vi "MainV1.vi"() -> ()   [LabVIEW 2010]
uses:
  <vilib>/Instr/_visa.llb/VISA Set IO Buffer Mask.ctl
  <vilib>/Instr/_visa.llb/VISA Flush IO Buffer Mask.ctl
  GlobalVar.vi
  <vilib>/Instr/_visa.llb/VISA Configure Serial Port (Instr).vi
panel:
  out "LongToSend":u8
  out "TypeToSend":u8
  out "DataToSend":u8[](array[numeric])
  out "Frequency":dbl
  out "Enum":T1(ring)
  out "error":errorcluster
  out "error Connexion":errorcluster
  out "Stop main loop":bool
  in  "stop":bool
  in  "Tab Control":T2(tab)
  out "Comm_LEDTest":bool
  in  "Comm_TestConnection":bool
  in  "Comm_BaudRate":u32=9600 caption="Baud rate"
  in  "Comm_PortComm":refnum<visa-resource-name>="COM7" caption="Communication Port"
  in  "timeout (10sec)":u32=10000
  in  "Con_RefreshIntensity":bool caption="Bouton OK 12"
  in  "Con_RefreshRightTorque":bool caption="Bouton OK 12"
  out "Con_XYIntensity":cluster{"Y":dbl[], "Y":dbl[]}[](graph) caption="Intensity"
  out "Con_XYRightTorque":cluster{"Y":dbl[], "Y":dbl[]}[](graph) caption="Motor right Torque"
  in  "Con_RefreshLeftTorque":bool caption="Bouton OK 12"
  out "Con_XYLeftTorque":cluster{"Y":dbl[], "Y":dbl[]}[](graph) caption="Motor left Torque"
  out "Con_IntensityMax":bool caption="Max Intensity"
  out "Con_Intensity":string[][](array[string]) caption="Intensity (A)"
  out "Con_MotorRightTorque":string[][](array[string]) caption="Motor right Torque (N.m)"
  out "Con_MotorLeftTorque":string[][](array[string]) caption="Motor left Torque (N.m)"
  in  "Ana_RefreshBattery":bool caption="Bouton OK 12"
  out "Ana_XYBattery":cluster{"Y":dbl[], "Y":dbl[]}[](graph) caption="Motor left Torque"
  in  "Ana_RefreshHandlebar":bool caption="Bouton OK 12"
  out "Ana_XYHandlebar":cluster{"Y":dbl[], "Y":dbl[]}[](graph) caption="Motor left Torque"
  out "Ana_Battery":string[][](array[string]) caption="Battery"
  out "Ana_Handlebar":string[][](array[string]) caption="Handlebar"
  in  "Inc_RefreshAcceleration":bool caption="Bouton OK 12"
  out "Inc_XYAcceleration":cluster{"Y":dbl[], "Y":dbl[]}[](graph) caption="Motor left Torque"
  in  "Inc_RefreshVelocityRightMotor":bool caption="Bouton OK 12"
  out "Inc_XYVelocityRightMotor":cluster{"Y":dbl[], "Y":dbl[]}[](graph) caption="Motor left Torque"
  in  "Inc_RefreshVelocityLeftMotor":bool caption="Bouton OK 12"
  out "Inc_XYVelocityLeftMotor":cluster{"Y":dbl[], "Y":dbl[]}[](graph) caption="Motor left Torque"
  out "Inc_Acceleration":string[][](array[string]) caption="Acceleration"
  out "Inc_VelocityRightMotor":string[][](array[string]) caption="Velocity Right motor"
  out "Inc_VelocityLeftMotor":string[][](array[string]) caption="Velocity left motor"
  out "Other_AngularVelocity":string[][](array[string]) caption="Angular velocity"
  out "Other_AngleOUT":string[][](array[string]) caption="Angle Out of range"
  out "Other_SpeedSaturation":string[][](array[string]) caption="Speed saturation"
  out "Other_Distance":string[][](array[string]) caption="Distance"
  out "Other_Angle":string[][](array[string]) caption="Angle"
  out "Spe_XY":cluster{"Y":dbl[], "Y":dbl[]}[](graph) caption="Motor left Torque"
  in  "Spe_Time":dbl caption="Time"
  in  "Spe_SendAnalysis":bool caption="Send Analysis"
  in  "Spe_Frequency":dbl caption="Frequency"
  out "Spe_Liste":string(combo) caption="Type"
  in  "Config_VelocitySaturation":dbl caption="VelocitySaturation"
  in  "Config_Sendvelocitysaturation":bool caption="Set velocity saturation"
  out "Config_Ready":string caption="Ready"
  out "Config_CurrentState":string caption="Current state"
  in  "Config_SendReady":bool caption="Ready ?"
  in  "Config_SendCurrentState":bool caption="Current state ?"
  in  "Config_SendRestart":bool caption="Re Start system"
  in  "Config_SendSTOP":bool caption="STOP system"
  out "Config_tCoefKalman":dbl caption="tCoef Kalman"
  in  "Config_ReceiveKalman":bool
  in  "Config_SendCoefKalman":bool
  in  "Config_CoefKalman":dbl caption="Coef Kalman"
  in  "Config_SendCoefAcc":bool
  in  "Config_CoefAcc":dbl caption="Coef System Acc"
  out "Config_tCoefdir":dbl caption="tCoef direction"
  in  "Config_SendCoefDir":bool
  in  "Config_CoeffDir":dbl caption="Coeff dir"
  in  "Config_ReceiveCoefDir":bool
  out "Config_tD":dbl caption="tD"
  out "Config_tI":dbl caption="tI"
  out "Config_tK":dbl caption="tK"
  in  "Config_ReceiveD":bool caption="Bouton OK 6"
  in  "Config_ReceiveI":bool
  in  "Config_ReceiveK":bool
  in  "Config_SendD":bool
  in  "Config_SendI":bool
  in  "Config_SendK":bool
  in  "Config_D":dbl caption="D"
  in  "Config_I":dbl caption="I"
  in  "Config_K":dbl caption="K"
  in  "Config_SendPID":bool
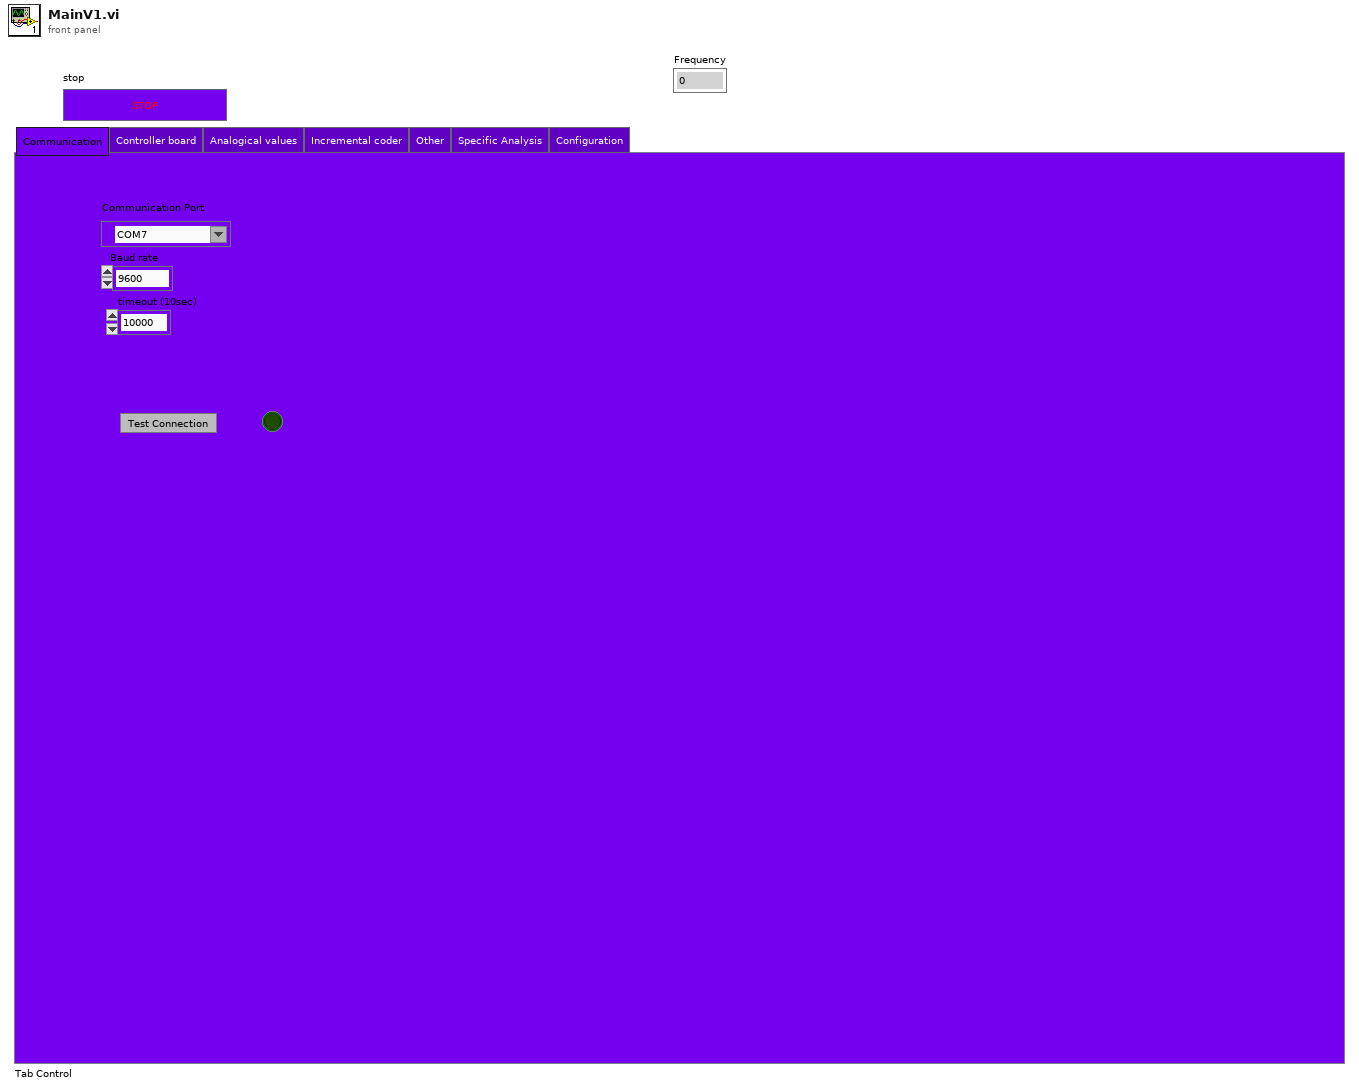
[diagram p1: front panel]
types:
  T1 = enum16{"Comm_TestConnection", "Con_RefreshLeftTorque", "Con_RefreshRightTorque", "Con_RefreshIntensity", "Ana_RefreshBattery", "Ana_RefreshHandlebar", "Inc_RefreshVelocityLeftMotor", "Inc_RefreshVelocityRightMotor", "Inc-RefreshAcceleration", "Spe_SendAnalysis", "Config_SendK", "Config_ReceiveK", "Config_SendD", "Config_ReceiveD", "Config_SendI", "Config_ReceiveI", "Config_SendCoefDir", "Config_ReceiveCoefDir", "Config_SendPID", "Config_SendCoefAcc", "Config_SendCoefKalman", "Config_ReceiveKalman", "Config_SendSTOP", "Config_SendRestart", "Config_SendCurrentState", "Config_SendReady", "Config_Sendvelocitysaturation", "Waiting"}
  T2 = enum32{"Communication", "Controller board", "Analogical values", "Incremental coder", "Other", "Specific Analysis", "Configuration"}
  T3 = typedef "VISA Set IO Buffer Mask.ctl" = u16
  T4 = typedef "VISA Flush IO Buffer Mask.ctl" = u16
  T5 = enum8{"Enabled", "Disabled", "Disabled and Grayed Out"}
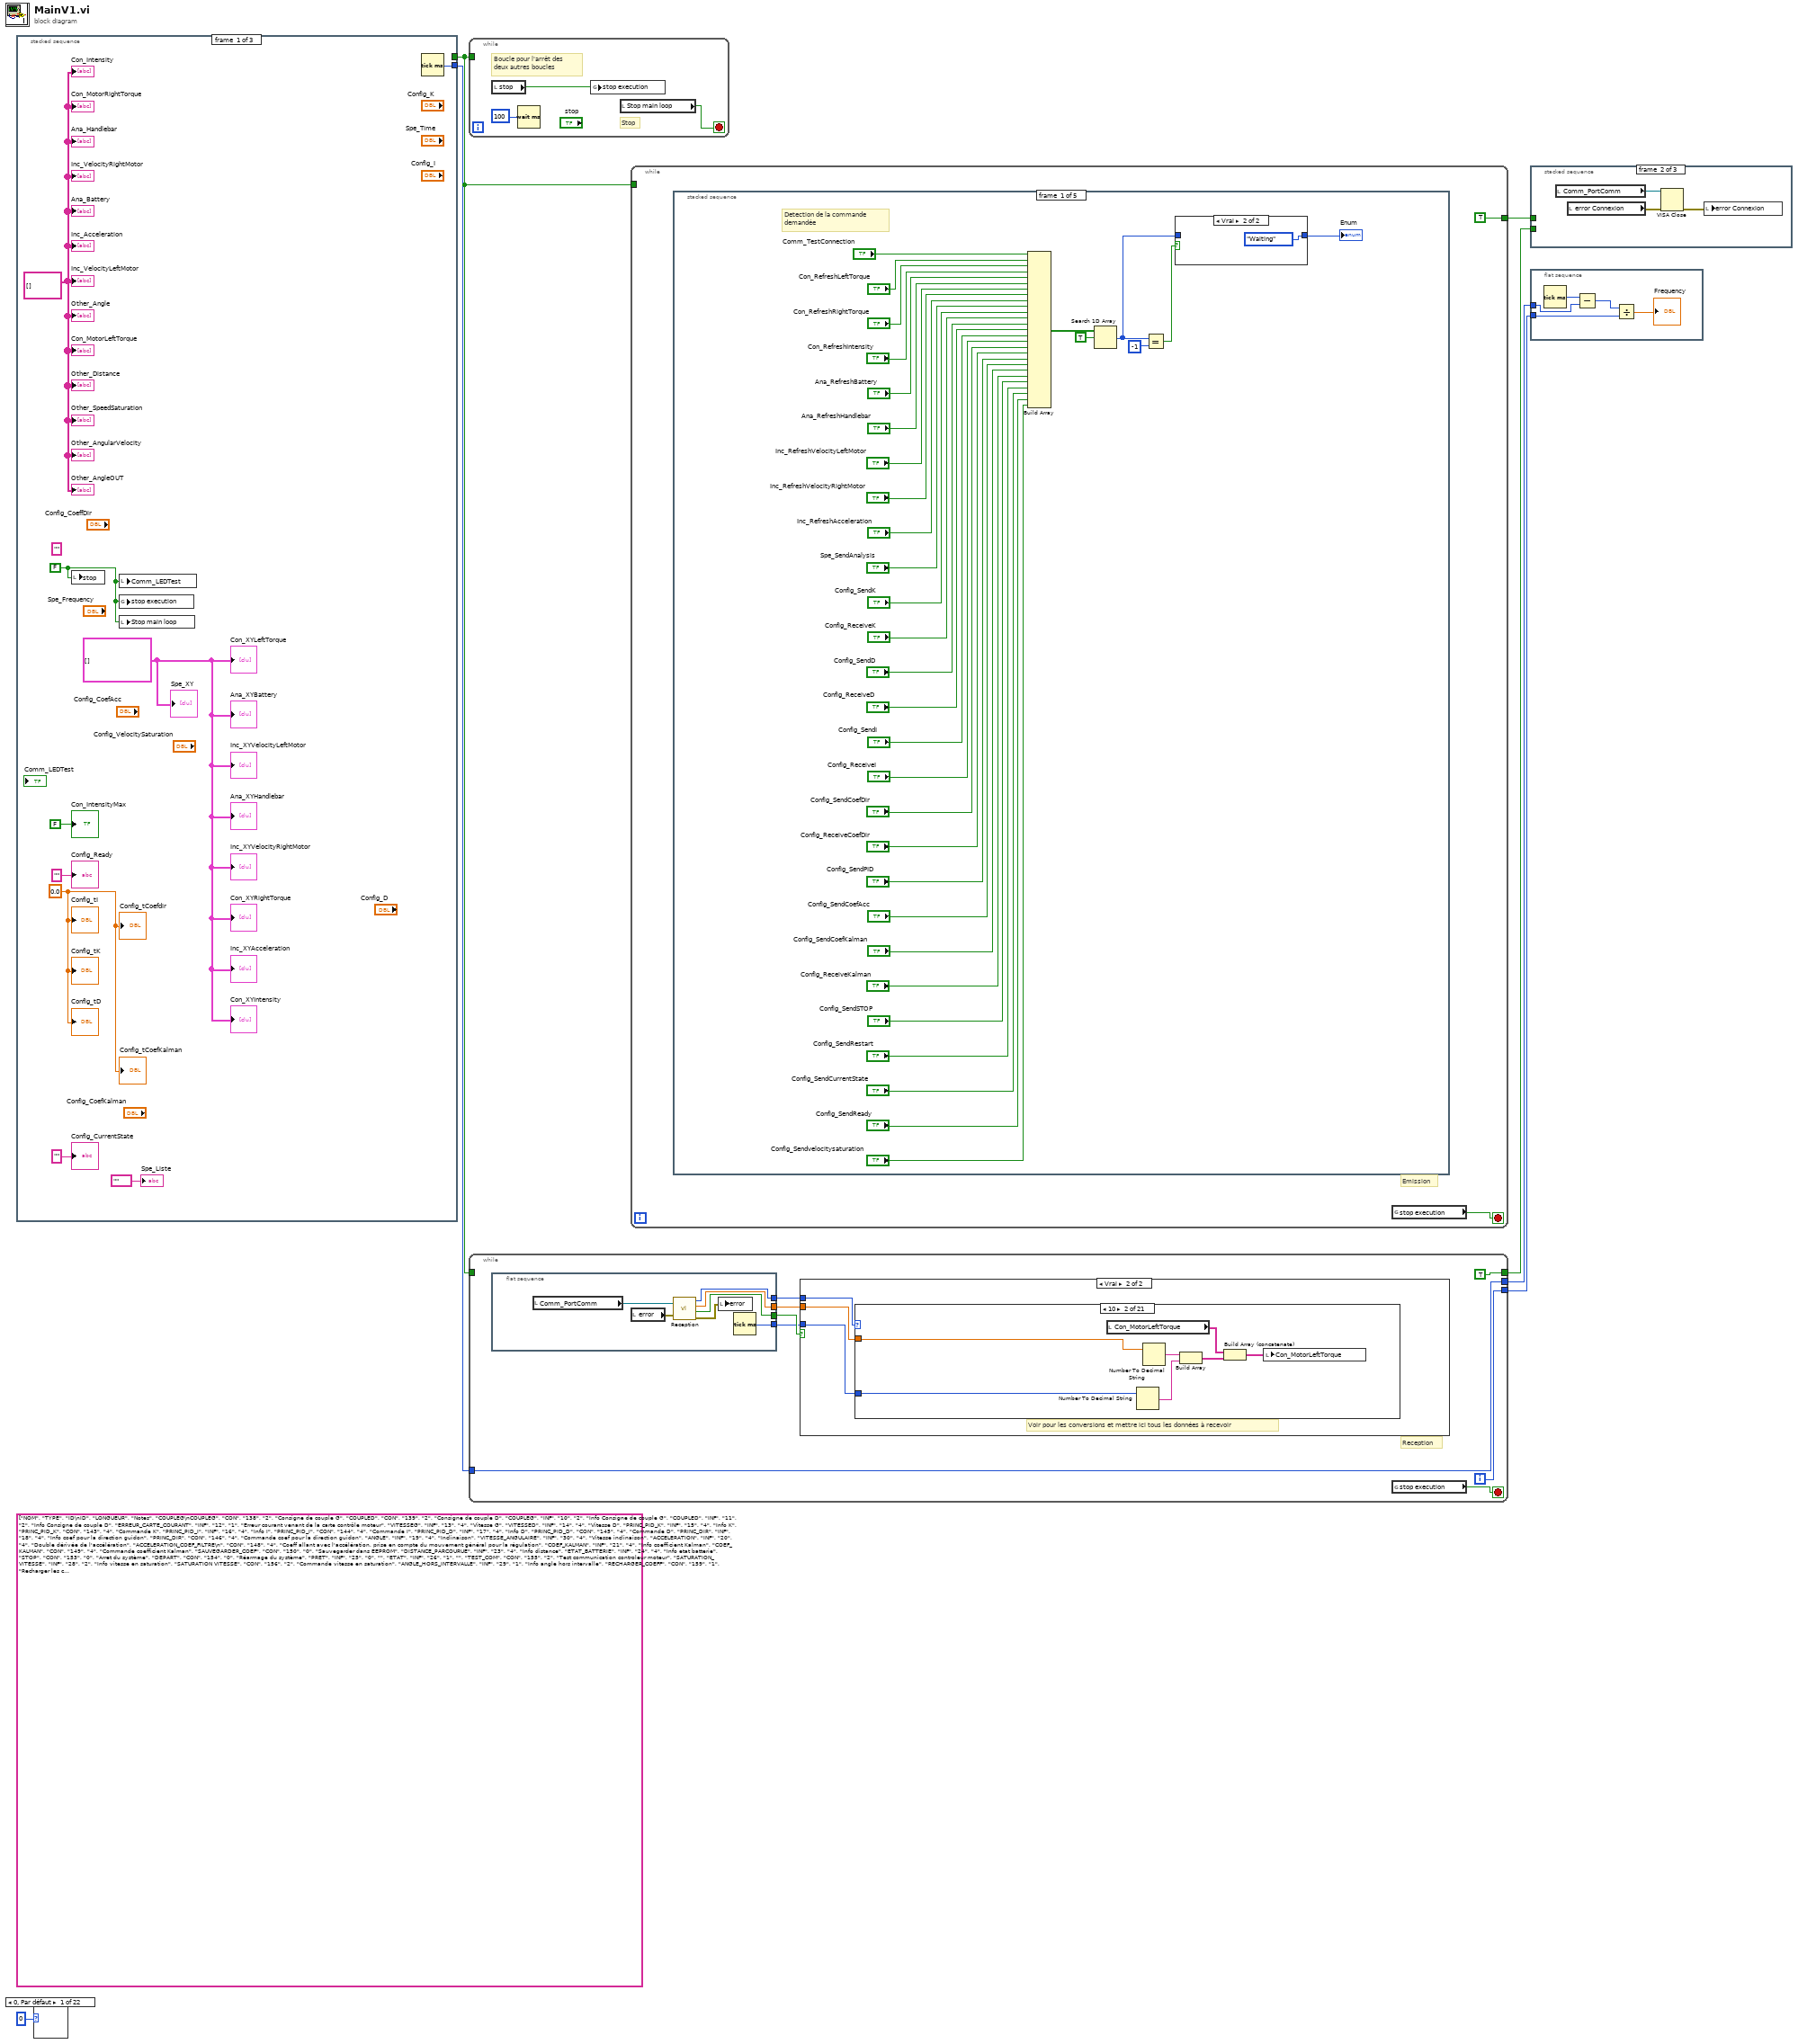
[diagram p0: block diagram]
diagram:
  (unwired) string[][] [["NOM", "TYPE", "ID\nID", "LONGUEUR", "Notes"], ["COUPLEG\nCOUPLEG", "CON", "138", "2", "Consigne de couple G"], ["COUPLED", "CON", "139", "2", "Consigne de couple D"], ["COUPLEG", "INF", "10", "2", "Info Consigne de couple G"], ["COUPLED", "INF", "11", "2", "Info Consigne de couple D"], ["ERREUR_CARTE_COURANT", "INF", "12", "1", "Erreur courant venant de la carte contrôle moteur"], ["VITESSEG", "INF", "13", "4", "Vitesse G"], ["VITESSED", "INF", "14", "4", "Vitesse D"], ["PRINC_PID_K", "INF", "15", "4", "Info K"], ["PRINC_PID_K", "CON", "143", "4", "Commande K"], ["PRINC_PID_I", "INF", "16", "4", "Info I"], ["PRINC_PID_I", "CON", "144", "4", "Commande I"], ["PRINC_PID_D", "INF", "17", "4", "Info D"], ["PRINC_PID_D", "CON", "145", "4", "Commande D"], ["PRINC_DIR", "INF", "18", "4", "Info coef pour la direction guidon"], ["PRINC_DIR", "CON", "146", "4", "Commande coef pour la direction guidon"], ["ANGLE", "INF", "19", "4", "Inclinaison"], ["VITESSE_ANGULAIRE", "INF", "30", "4", "Vitesse inclinaison"], ["ACCELERATION", "INF", "20", "4", "Double dérivée de l'accélération"], ["ACCELERATION_COEF_FILTRE\n", "CON", "148", "4", "Coeff allant avec l'accélération, prise en compte du mouvement général pour la régulation"], ["COEF_KALMAN", "INF", "21", "4", "Info coefficient Kalman"], ["COEF_KALMAN", "CON", "149", "4", "Commande coefficient Kalman"], ["SAUVEGARDER_COEF", "CON", "150", "0", "Sauvegarder dans EEPROM"], ["DISTANCE_PARCOURUE", "INF", "23", "4", "Info distance"], ["ETAT_BATTERIE", "INF", "24", "4", "Info etat batterie"], ["STOP", "CON", "153", "0", "Arret du système"], ["DEPART", "CON", "154", "0", "Réarmage du système"], ["PRET", "INF", "25", "0", ""], ["ETAT", "INF", "26", "1", ""], ["TEST_COM", "CON", "155", "2", "Test communication controleur moteur"], ["SATURATION_VITESSE", "INF", "28", "2", "Info vitesse en saturation"], ["SATURATION VITESSE", "CON", "156", "2", "Commande vitesse en saturation"], ["ANGLE_HORS_INTERVALLE", "INF", "29", "1", "Info angle hors intervalle"], ["RECHARGER_COEFF", "CON", "159", "1", "Recharger les coeff"]]
  n1 = stacked-sequence {
    tunnel: [_ _ TRUE] -> w7
    tunnel: [w15 _ _] -> w3
    frame #0 {
      w11 = 0.0 ("Config_tK")
      (unwired) "" ("Comm_Reception")
      w9 = cluster{"Y":dbl[], "Y":dbl[]}[] [] ("Ana_XYHandlebar 3")
      w8 = string[][] [] ("Velocity motor left")
      w16 = FALSE ("Comm_LEDTest")
      n2 = local write "stop"(w16) -> ()
      n3 = local write "Comm_LEDTest"(w16) -> ()
      n4 = global write "GlobalVar.vi" "stop execution"(w16) -> ()
      n5 = local write "Stop main loop"(w16) -> ()
      n6 = Tick Count (ms)() -> (millisecond timer value=w15:u32)
      "Con_IntensityMax" <- FALSE ("Con_IntensityMax")
      "Config_tK" <- w11
      "Config_tI" <- w11
      "Config_tD" <- w11
      "Config_tCoefdir" <- w11
      "Inc_Acceleration" <- w8
      "Config_tCoefKalman" <- w11
      "Other_Angle" <- w8
      "Config_CurrentState" <- "" ("Config_CurrentState")
      "Config_Ready" <- "" ("Config_Ready")
      "Other_SpeedSaturation" <- w8
      "Other_AngleOUT" <- w8
      "Other_Distance" <- w8
      "Ana_XYHandlebar" <- w9
      "Ana_XYBattery" <- w9
      "Inc_XYVelocityLeftMotor" <- w9
      "Inc_XYVelocityRightMotor" <- w9
      "Inc_XYAcceleration" <- w9
      "Spe_XY" <- w9
      "Con_MotorLeftTorque" <- w8
      "Con_MotorRightTorque" <- w8
      "Con_Intensity" <- w8
      "Inc_VelocityLeftMotor" <- w8
      "Inc_VelocityRightMotor" <- w8
      "Spe_Liste" <- "" ("Spe_Liste")
      "Ana_Handlebar" <- w8
      "Ana_Battery" <- w8
      "Con_XYRightTorque" <- w9
      "Con_XYIntensity" <- w9
      "Con_XYLeftTorque" <- w9
      "Other_AngularVelocity" <- w8
    }
    frame #1 {
      w18 = T3 48 items=["Buffer d'entrées (E/S)"=16, "Buffer de sorties (E/S)"=32, "Buffer d'entrées et de sorties (E/S)"=48] ("Mask")
      w22 = T4 16 items=["Vider le buffer d'entrées"=16, "Écrire le buffer de sorties sur le périphérique"=32, "Vider le buffer d'entrées (Pas d'E/S)"=64, "Vider le buffer de sorties"=128] ("Mask")
      w26 = u16 0 items=["None"=0, "XON/XOFF"=1, "RTS/CTS"=2, "DTR/DSR"=4] ("flow control")
      w27 = u16 10 items=["1.0"=10, "1.5"=15, "2.0"=20] ("stop bits")
      w29 = u16 0 items=["None", "Odd", "Even", "Mark", "Space"] ("parity")
      # "Initial"
      n7 = local write "Tab Control"(T2."Communication" ("Tab Control")) -> ()
      n8 = call-poly "VISA Configure Serial Port"("VISA resource name"="Comm_PortComm", "timeout (10sec)"="timeout (10sec)", "baud rate (9600)"="Comm_BaudRate", "data bits (8)"=u16 8 ("data bits"), "parity (0:none)"=w29, "stop bits (10: 1 bit)"=w27, "flow control (0:none)"=w26) -> ("VISA resource name out"=w23:refnum<visa-resource-name>, "error out"=w20:errorcluster)  [unwired: 2 in, 5 out]
      "error Connexion" <- w20
      "error" <- w20
      n9 = VISA Set I/O Buffer Size(VISA resource name=w23, mask (16)=w18, size (4096)=u32 524288 ("taille (4096)"), error in (no error)=w20) -> (VISA resource name out=w21:refnum<visa-resource-name>, error out=w19:errorcluster)
      n10 = VISA Flush I/O Buffer(VISA resource name=w21, mask (16)=w22, error in (no error)=w19) -> ()  [unwired: 2 out]
    }
    frame #2 {
      # "OK Initialisation"
    }
  }
  n11 = case shown="0, Par défaut" 0 {
    frame 0, Default {
    }
    frame 10 {
    }
    frame 11 {
    }
    frame 12 {
    }
    frame 13 {
    }
    frame 14 {
    }
    frame 15 {
    }
    frame 16 {
    }
    frame 17 {
    }
    frame 18 {
    }
    frame 19 {
    }
    frame 20 {
    }
    frame 21 {
    }
    frame 22 {
    }
    frame 23 {
    }
    frame 24 {
    }
    frame 25 {
    }
    frame 26 {
    }
    frame 27 {
    }
    frame 28 {
    }
    frame 29 {
    }
    frame 30 {
    }
  }
  n12 = while {
    tunnel: w7 -> [_]
    stop <- w34 stop-if-true
    # "Boucle pour l'arrêt des \ndeux autres boucles"
    # "Stop"
    n13 = local read "stop"() -> (w35:bool)
    n14 = Wait (ms)(milliseconds to wait=u32 100) -> ()  [unwired: 1 out]
    n15 = global write "GlobalVar.vi" "stop execution"(w35) -> ()
    n16 = local read "Stop main loop"() -> (w34:bool)
  }
  n17 = while {
    tunnel: w7 -> [_]
    tunnel: [TRUE] -> w6
    tunnel: w3 -> [w36]
    tunnel: [w37] -> w2
    tunnel: [w36] -> w1
    i -> [w37]
    stop <- w42 stop-if-true
    # "Reception"
    n18 = flat-sequence {
      tunnel: [w48] -> w41
      tunnel: [w47] -> w40
      tunnel: [w46] -> w39
      tunnel: [w45] -> w38
      frame #0 {
        n19 = local read "Comm_PortComm"() -> (w50:refnum<visa-resource-name>)
        n20 = local read "error"() -> (w49:errorcluster)
        n21 = call "Reception.vi"("entrée d'erreur (pas d'erreur)"=w49, "Nom de ressource VISA"=w50) -> ("Sortie d'erreur"=w44:errorcluster, "Checksum OK?"=w48:bool, "Data"=w46:dbl, "ID byte"=w47:i32)
        n22 = local write "error"(w44) -> ()
        n23 = Tick Count (ms)() -> (millisecond timer value=w45:u32)
      }
    }
    n24 = case shown="Vrai" w41 {
      tunnel: w40 -> [_ w53]
      tunnel: w39 -> [_ w52]
      tunnel: w38 -> [_ w51]
      frame False {
      }
      frame True {
        # "Voir pour les conversions et mettre ici tous les données à recevoir"
        n25 = case shown="10" w53 {
          tunnel: w52 -> [_ w59 w62 w69 w71 w79 w86 w87 w88 w89 w90 w99 w106 w108 w116 _ _ _ w124 _ w132]
          tunnel: w51 -> [_ w58 w61 _ w72 w80 _ _ _ _ w91 w98 _ w107 w115 _ _ _ w123 _ w131]
          frame 0, Default {
          }
          frame 10 {
            n26 = local read "Con_MotorLeftTorque"() -> (w60:string[][])
            n27 = Number To Decimal String(number=w58) -> (decimal integer string=w56:string)  [unwired: 1 in]
            n28 = Number To Decimal String(number=w59) -> (decimal integer string=w57:string)  [unwired: 1 in]
            n29 = Build Array(w57, w56) -> (w55:string[])
            n30 = Build Array (concatenate)(w60, w55) -> (w54:string[][])
            n31 = local write "Con_MotorLeftTorque"(w54) -> ()
          }
          frame 11 {
            n32 = local read "Con_MotorRightTorque"() -> (w67:string[][])
            n33 = Number To Decimal String(number=w61) -> (decimal integer string=w65:string)  [unwired: 1 in]
            n34 = Number To Decimal String(number=w62) -> (decimal integer string=w66:string)  [unwired: 1 in]
            n35 = Build Array(w66, w65) -> (w64:string[])
            n36 = Build Array (concatenate)(w67, w64) -> (w63:string[][])
            n37 = local write "Con_MotorRightTorque"(w63) -> ()
          }
          frame 12 {
            n38 = Not Equal To 0?(x=w69) -> (x != 0?=w68:bool)
            n39 = local write "Con_IntensityMax"(w68) -> ()
          }
          frame 13 {
            n40 = local read "Inc_VelocityLeftMotor"() -> (w77:string[][])
            n41 = Number To Decimal String(number=w72) -> (decimal integer string=w75:string)  [unwired: 1 in]
            n42 = Number To Exponential String(number=w71, precision (6)=i16 3 ("précision (6)")) -> (E-format string=w76:string)  [unwired: 2 in]
            n43 = Build Array(w76, w75) -> (w74:string[])
            n44 = Build Array (concatenate)(w77, w74) -> (w73:string[][])
            n45 = local write "Inc_VelocityLeftMotor"(w73) -> ()
          }
          frame 14 {
            n46 = local read "Inc_VelocityRightMotor"() -> (w85:string[][])
            n47 = Number To Decimal String(number=w80) -> (decimal integer string=w83:string)  [unwired: 1 in]
            n48 = Number To Exponential String(number=w79, precision (6)=i16 3 ("précision (6)")) -> (E-format string=w84:string)  [unwired: 2 in]
            n49 = Build Array(w84, w83) -> (w82:string[])
            n50 = Build Array (concatenate)(w85, w82) -> (w81:string[][])
            n51 = local write "Inc_VelocityRightMotor"(w81) -> ()
          }
          frame 15 {
            n52 = local write "Config_tK"(w86) -> ()
          }
          frame 16 {
            n53 = local write "Config_tI"(w87) -> ()
          }
          frame 17 {
            n54 = local write "Config_tD"(w88) -> ()
          }
          frame 18 {
            n55 = local write "Config_tCoefdir"(w89) -> ()
          }
          frame 19 {
            n56 = Number To Decimal String(number=w91) -> (decimal integer string=w95:string)  [unwired: 1 in]
            n57 = Number To Exponential String(number=w90, precision (6)=i16 3 ("précision (6)")) -> (E-format string=w96:string)  [unwired: 2 in]
            n58 = local read "Other_Angle"() -> (w97:string[][])
            n59 = Build Array(w96, w95) -> (w94:string[])
            n60 = Build Array (concatenate)(w97, w94) -> (w93:string[][])
            n61 = local write "Other_Angle"(w93) -> ()
          }
          frame 20 {
            n62 = local read "Inc_Acceleration"() -> (w105:string[][])
            n63 = Number To Decimal String(number=w98) -> (decimal integer string=w103:string)  [unwired: 1 in]
            n64 = Number To Exponential String(number=w99, precision (6)=i16 3 ("précision (6)")) -> (E-format string=w104:string)  [unwired: 2 in]
            n65 = Build Array(w104, w103) -> (w102:string[])
            n66 = Build Array (concatenate)(w105, w102) -> (w101:string[][])
            n67 = local write "Inc_Acceleration"(w101) -> ()
          }
          frame 21 {
            n68 = local write "Config_tCoefKalman"(w106) -> ()
          }
          frame 23 {
            n69 = Number To Decimal String(number=w107) -> (decimal integer string=w112:string)  [unwired: 1 in]
            n70 = local read "Other_Distance"() -> (w114:string[][])
            n71 = Number To Exponential String(number=w108, precision (6)=i16 3 ("précision (6)")) -> (E-format string=w113:string)  [unwired: 2 in]
            n72 = Build Array(w113, w112) -> (w111:string[])
            n73 = Build Array (concatenate)(w114, w111) -> (w110:string[][])
            n74 = local write "Other_Distance"(w110) -> ()
          }
          frame 24 {
            n75 = Number To Decimal String(number=w115) -> (decimal integer string=w120:string)  [unwired: 1 in]
            n76 = Number To Exponential String(number=w116, precision (6)=i16 3 ("précision (6)")) -> (E-format string=w121:string)  [unwired: 2 in]
            n77 = local read "Ana_Battery"() -> (w122:string[][])
            n78 = Build Array(w121, w120) -> (w119:string[])
            n79 = Build Array (concatenate)(w122, w119) -> (w118:string[][])
            n80 = local write "Ana_Battery"(w118) -> ()
          }
          frame 25 {
          }
          frame 26 {
          }
          frame 27 {
          }
          frame 28 {
            n81 = local read "Other_SpeedSaturation"() -> (w130:string[][])
            n82 = Number To Decimal String(number=w123) -> (decimal integer string=w128:string)  [unwired: 1 in]
            n83 = Number To Exponential String(number=w124, precision (6)=i16 3 ("précision (6)")) -> (E-format string=w129:string)  [unwired: 2 in]
            n84 = Build Array(w129, w128) -> (w127:string[])
            n85 = Build Array (concatenate)(w130, w127) -> (w126:string[][])
            n86 = local write "Other_SpeedSaturation"(w126) -> ()
          }
          frame 29 {
          }
          frame 30 {
            n87 = local read "Other_AngularVelocity"() -> (w138:string[][])
            n88 = Number To Decimal String(number=w131) -> (decimal integer string=w136:string)  [unwired: 1 in]
            n89 = Number To Exponential String(number=w132, precision (6)=i16 3 ("précision (6)")) -> (E-format string=w137:string)  [unwired: 2 in]
            n90 = Build Array(w137, w136) -> (w135:string[])
            n91 = Build Array (concatenate)(w138, w135) -> (w134:string[][])
            n92 = local write "Other_AngularVelocity"(w134) -> ()
          }
        }
      }
    }
    n93 = global read "GlobalVar.vi" "stop execution"() -> (w42:bool)
  }
  n94 = while {
    tunnel: w7 -> [_]
    tunnel: [TRUE] -> w5
    stop <- w139 stop-if-true
    # "Emission"
    n95 = stacked-sequence {
      frame #0 {
        # "Detection de la commande\ndemandée"
        n96 = Build Array("Comm_TestConnection", "Con_RefreshLeftTorque", "Con_RefreshRightTorque", "Con_RefreshIntensity", "Ana_RefreshBattery", "Ana_RefreshHandlebar", "Inc_RefreshVelocityLeftMotor", "Inc_RefreshVelocityRightMotor", "Inc_RefreshAcceleration", "Spe_SendAnalysis", "Config_SendK", "Config_ReceiveK", "Config_SendD", "Config_ReceiveD", "Config_SendI", "Config_ReceiveI", "Config_SendCoefDir", "Config_ReceiveCoefDir", "Config_SendPID", "Config_SendCoefAcc", "Config_SendCoefKalman", "Config_ReceiveKalman", "Config_SendSTOP", "Config_SendRestart", "Config_SendCurrentState", "Config_SendReady", "Config_Sendvelocitysaturation") -> (w173:bool[])
        n97 = Search 1D Array(1D array=w173, element=TRUE) -> (index of element=w169:i32)  [unwired: 1 in]
        n98 = Equal?(x=w169, y=-1) -> (x = y?=w171:bool)
        n99 = case shown="Vrai" w171 {
          tunnel: [w174 T1."Waiting" ("Enum 2")] -> w170
          tunnel: w169 -> [w174 _]
          frame False {
          }
          frame True {
          }
        }
        "Enum" <- w170
      }
      frame #1 {
        n100 = local read "Enum"() -> (w177:T1)
        n101 = Not Equal?(x=w177, y=T1."Waiting") -> (x != y?=w178:bool)
        n102 = case shown="Faux" w178 {
          frame False {
          }
          frame True {
            w179 = T5."Disabled and Grayed Out" ("Disabled")
            # "Disable all commands"
            n103 = property on="Spe_SendAnalysis" class="Bool"("DisabledEnum"=w179) -> ()  [unwired: 2 in, 2 out]
            n104 = property on="Comm_TestConnection" class="Bool"("DisabledEnum"=w179) -> ()  [unwired: 2 in, 2 out]
          }
        }
      }
      frame #2 {
        # "Traitement de la commande,\nboucles pour des mesures avec création \nde la trame série,\nautre pour la configuration"
        n105 = local read "Enum"() -> (w180:T1)
        n106 = case shown="\"Con_RefreshLeftTorque\"" w180 {
          frame "Comm_TestConnection" {
            n107 = One Button Dialog(message="Not available.") -> ()  [unwired: 1 in, 1 out]
          }
          frame "Con_RefreshRightTorque" {
            n108 = local read "Con_MotorRightTorque"() -> (w183:string[][])
            n109 = call "TableToXYGraph.vi"("Input Table"=w183) -> ("XY Graph"=w182:cluster{"Y":dbl[], "Y":dbl[]}[])
            n110 = local write "Con_XYRightTorque"(w182) -> ()
          }
          frame "Con_RefreshIntensity" {
            n111 = local read "Con_Intensity"() -> (w185:string[][])
            n112 = call "TableToXYGraph.vi"("Input Table"=w185) -> ("XY Graph"=w184:cluster{"Y":dbl[], "Y":dbl[]}[])
            n113 = local write "Con_XYIntensity"(w184) -> ()
          }
          frame "Ana_RefreshBattery" {
            n114 = local read "Ana_Battery"() -> (w187:string[][])
            n115 = call "TableToXYGraph.vi"("Input Table"=w187) -> ("XY Graph"=w186:cluster{"Y":dbl[], "Y":dbl[]}[])
            n116 = local write "Ana_XYBattery"(w186) -> ()
          }
          frame "Ana_RefreshHandlebar" {
            n117 = local read "Ana_Handlebar"() -> (w189:string[][])
            n118 = call "TableToXYGraph.vi"("Input Table"=w189) -> ("XY Graph"=w188:cluster{"Y":dbl[], "Y":dbl[]}[])
            n119 = local write "Ana_XYHandlebar"(w188) -> ()
          }
          frame "Inc_RefreshVelocityLeftMotor" {
            n120 = local read "Inc_VelocityLeftMotor"() -> (w191:string[][])
            n121 = call "TableToXYGraph.vi"("Input Table"=w191) -> ("XY Graph"=w190:cluster{"Y":dbl[], "Y":dbl[]}[])
            n122 = local write "Inc_XYVelocityLeftMotor"(w190) -> ()
          }
          frame "Inc_RefreshVelocityRightMotor" {
            n123 = local read "Inc_VelocityRightMotor"() -> (w193:string[][])
            n124 = call "TableToXYGraph.vi"("Input Table"=w193) -> ("XY Graph"=w192:cluster{"Y":dbl[], "Y":dbl[]}[])
            n125 = local write "Inc_XYVelocityRightMotor"(w192) -> ()
          }
          frame "Inc-RefreshAcceleration" {
            n126 = local read "Inc_Acceleration"() -> (w195:string[][])
            n127 = call "TableToXYGraph.vi"("Input Table"=w195) -> ("XY Graph"=w194:cluster{"Y":dbl[], "Y":dbl[]}[])
            n128 = local write "Inc_XYAcceleration"(w194) -> ()
          }
          frame "Spe_SendAnalysis" {
            n129 = One Button Dialog(message="Not available.") -> ()  [unwired: 1 in, 1 out]
          }
          frame "Config_SendK" {
            w200 = u8[] []  # type U8
            n130 = local write "LongToSend"(u8 4 ("LongToSend")) -> ()
            n131 = local write "TypeToSend"(u8 143 ("TypeToSend")) -> ()
            n132 = local read "Config_K"() -> (w201:dbl)
            n133 = Type Cast(type=w200, x=w201) -> (*(type *) &x=w199:u8[])
            n134 = local write "DataToSend"(w199) -> ()
          }
          frame "Config_ReceiveK" {
            n135 = One Button Dialog(message="Not available.") -> ()  [unwired: 1 in, 1 out]
          }
          frame "Config_SendD" {
            n136 = One Button Dialog(message="Not available.") -> ()  [unwired: 1 in, 1 out]
          }
          frame "Config_ReceiveD" {
            n137 = One Button Dialog(message="Not available.") -> ()  [unwired: 1 in, 1 out]
          }
          frame "Config_SendI" {
            n138 = One Button Dialog(message="Not available.") -> ()  [unwired: 1 in, 1 out]
          }
          frame "Config_ReceiveI" {
            n139 = One Button Dialog(message="Not available.") -> ()  [unwired: 1 in, 1 out]
          }
          frame "Config_SendCoefDir" {
            n140 = One Button Dialog(message="Not available.") -> ()  [unwired: 1 in, 1 out]
          }
          frame "Config_ReceiveCoefDir" {
            n141 = One Button Dialog(message="Not available.") -> ()  [unwired: 1 in, 1 out]
          }
          frame "Config_SendPID" {
            n142 = One Button Dialog(message="Not available.") -> ()  [unwired: 1 in, 1 out]
          }
          frame "Config_SendCoefAcc" {
            n143 = One Button Dialog(message="Not available.") -> ()  [unwired: 1 in, 1 out]
          }
          frame "Config_SendCoefKalman" {
            n144 = One Button Dialog(message="Not available.") -> ()  [unwired: 1 in, 1 out]
          }
          frame "Config_ReceiveKalman" {
            n145 = One Button Dialog(message="Not available.") -> ()  [unwired: 1 in, 1 out]
          }
          frame "Config_SendSTOP" {
            n146 = One Button Dialog(message="Not available.") -> ()  [unwired: 1 in, 1 out]
          }
          frame "Config_SendRestart" {
            n147 = One Button Dialog(message="Not available.") -> ()  [unwired: 1 in, 1 out]
          }
          frame "Config_SendCurrentState" {
            n148 = One Button Dialog(message="Not available.") -> ()  [unwired: 1 in, 1 out]
          }
          frame "Config_SendReady" {
            n149 = One Button Dialog(message="Not available.") -> ()  [unwired: 1 in, 1 out]
          }
          frame "Config_Sendvelocitysaturation" {
            n150 = One Button Dialog(message="Not available.") -> ()  [unwired: 1 in, 1 out]
          }
          frame "Waiting", Default {
          }
          frame "Con_RefreshLeftTorque" {
            n151 = local read "Con_MotorLeftTorque"() -> (w219:string[][])
            n152 = call "TableToXYGraph.vi"("Input Table"=w219) -> ("XY Graph"=w218:cluster{"Y":dbl[], "Y":dbl[]}[])
            n153 = local write "Con_XYLeftTorque"(w218) -> ()
          }
        }
      }
      frame #3 {
        # "Envoyer la trame"
        n154 = local read "Comm_PortComm"() -> (w220:refnum<visa-resource-name>)
        n155 = local read "TypeToSend"() -> (w222:u8)
        n156 = local read "DataToSend"() -> (w221:u8[])
        n157 = local read "error"() -> (w223:errorcluster)
        n158 = call "Send.vi"("entrée d'erreur (pas d'erreur)"=w223, "tableau d'octets non signés"=w221, "Type"=w222, "Nom de ressource VISA"=w220) -> ("sortie d'erreur"=w224:errorcluster)
        n159 = local write "error"(w224) -> ()
      }
      frame #4 {
        w225 = T5."Enabled" ("Disabled")
        # "Disable all commands"
        # "Activate all commands"
        n160 = property on="Spe_SendAnalysis" class="Bool"("DisabledEnum"=w225) -> ()  [unwired: 2 in, 2 out]
        n161 = property on="Comm_TestConnection" class="Bool"("DisabledEnum"=w225) -> ()  [unwired: 2 in, 2 out]
      }
    }
    n162 = global read "GlobalVar.vi" "stop execution"() -> (w139:bool)
  }
  n163 = stacked-sequence {
    tunnel: w6 -> [_ _ _]
    tunnel: w5 -> [w226 _ _]
    frame #0 {
      # "Finalisation"
      "Stop main loop" <- w226
    }
    frame #1 {
      n164 = local read "Comm_PortComm"() -> (w229:refnum<visa-resource-name>)
      n165 = local read "error Connexion"() -> (w228:errorcluster)
      n166 = VISA Close(VISA resource name=w229, error in (no error)=w228) -> (error out=w227:errorcluster)
      n167 = local write "error Connexion"(w227) -> ()
    }
    frame #2 {
      n168 = local read "error Connexion"() -> (w232:errorcluster)
      n169 = local read "error"() -> (w231:errorcluster)
      n170 = Merge Errors(w231, w232) -> (w230:errorcluster)
      n171 = call <vilib>:"Simple Error Handler.vi"("error in (no error)"=w230) -> ()  [unwired: 4 in, 5 out]
    }
  }
  n172 = flat-sequence {
    tunnel: w2 -> [w234]
    tunnel: w1 -> [w236]
    frame #0 {
      n173 = Tick Count (ms)() -> (millisecond timer value=w237:u32)
      n174 = Subtract(x=w237, y=w236) -> (x-y=w235:u32)
      n175 = Divide(x=w235, y=w234) -> (x/y=→"Frequency":dbl)
    }
  }
